vi "Psychro Solver.vi"(7 "Incomplete Air Flow State":T1={"Flow Rate [CFM]"=0.0, "Pressure [psia]"=14.696, "Dry Bulb Temp [DegF]"=-460.0, "Wet Bulb Temp [DegF]"=-460.0, "Relative Humidity [%]"=-460.0, "Humidity Ratio [lbmv/lbma]"=-460.0, "Grains [Gr/lbma]"=-460.0, "Specific Volume [ft^3/lbma]"=-460.0, "Enthalpy [BTU/lbm]"=-460.0, "Dew Point [DegF]"=-460.0}) -> (8 "Complete Air Flow State":T1={"Flow Rate [CFM]"=0.0, "Pressure [psia]"=0.0, "Dry Bulb Temp [DegF]"=-460.0, "Wet Bulb Temp [DegF]"=-460.0, "Relative Humidity [%]"=-460.0, "Humidity Ratio [lbmv/lbma]"=-460.0, "Grains [Gr/lbma]"=-460.0, "Specific Volume [ft^3/lbma]"=-460.0, "Enthalpy [BTU/lbm]"=-460.0, "Dew Point [DegF]"=-460.0})   [LabVIEW 2020]
uses:
  Utilities/Air Flow State.ctl
  Utilities/Air Constants.vi
panel:
  out "2nd Property":dbl
  out "1st Property":dbl
  out "2nd Known Index":u16(ring)=2 items=["DB", "WB", "RH", "HR", "Gr", "Vol", "h", "Dp"]
  out "array w/ 1st \nproperty set to -460":dbl[](array[numeric])=[-460.0, -460.0, -460.0, -460.0, -200.0, -460.0, -460.0, -460.0]
  out "array w/ subset deleted":dbl[](array[numeric])=[-460.0, -460.0, -460.0, -460.0, -200.0, -460.0, -460.0, -460.0]
  out "1st Known Index":u16(ring) items=["DB", "WB", "RH", "HR", "Gr", "Vol", "h", "Dp"]
  # "Data was generated using the the \nkW Psychrometric Functions Library for Excel:\n\nhttps://www.kw-engineering.com/psychrometrics/"
  # "As of 6/3/21 - Program is completed and checked with the following\nnotes:\n\n* CANNOT Perform Look-up if the two variables entered are:\n     DB & h\n     DB & v\n      h & v\n\n     This is because the excel function used to generate the tables MUST \n      have DB as one of the inputs, and the function cannot accept v or h as an input.\n\n*  Program does not behave well if input is WB & h. On psych chart, these two variables\n    appear to be independent (parallel lines)\n\n*Program does not behave well if input is HR/Gr & DP. On psych chart, these two variables\n     appear to be independent"
  # "These cases return NaN"
  # "TO DO: \n\nFigure out how to make program work for remaining scenarios\n\nDocument error range (a quick spot check never returned a value with more than 1% error. \nChecked for combinations compatible with the TRANE HDPsyChart App [must input DB]. Situations \nnot compatible with that App were checked by eye with the app's psych chart. P = 14.696 psia only\npressure checked so far.)"
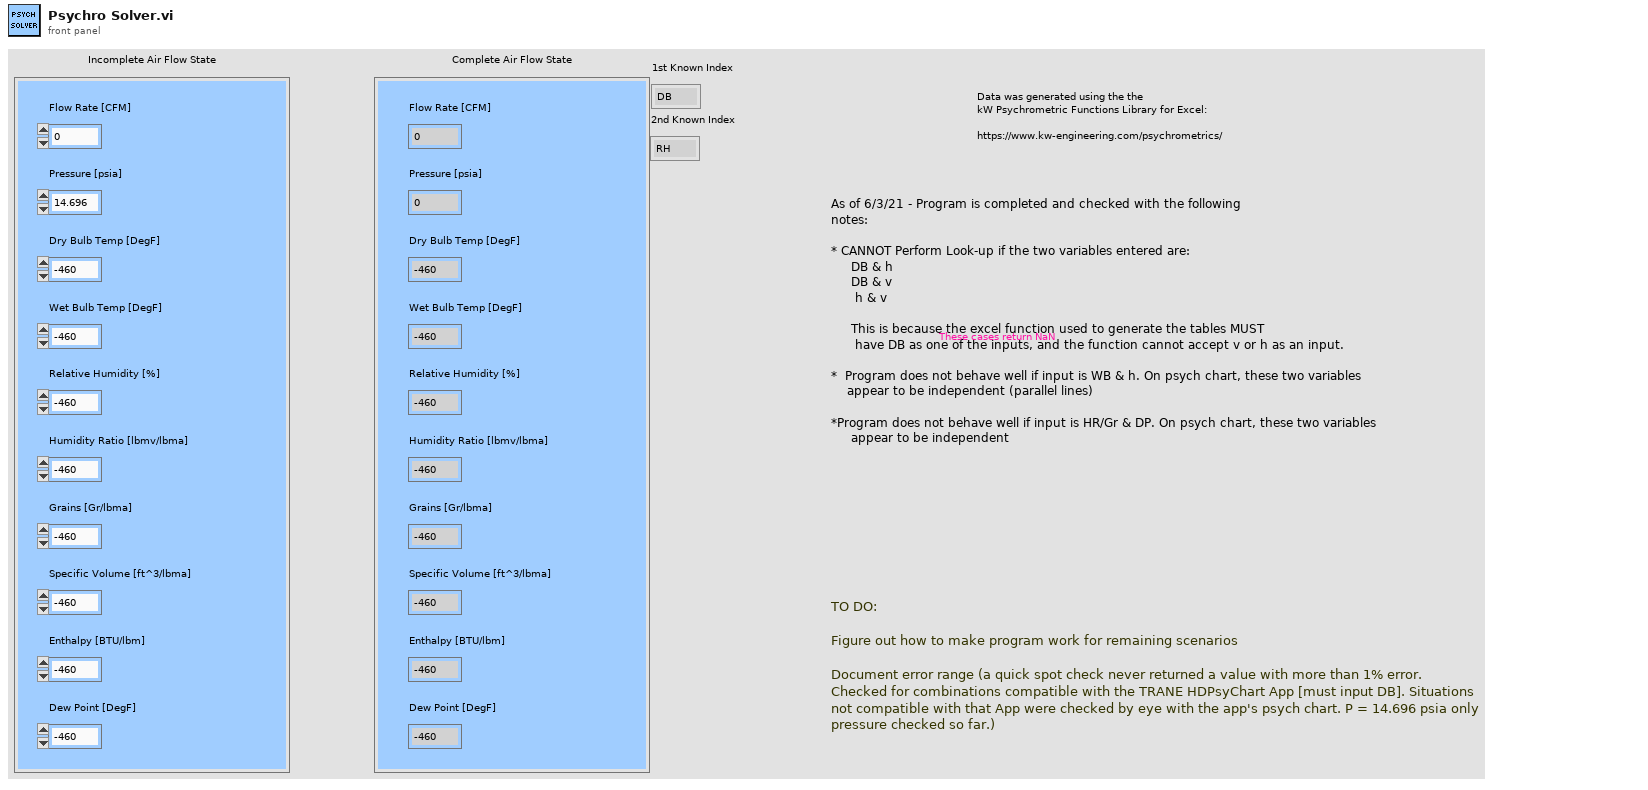
[diagram p1: front panel]
types:
  T1 = typedef "Air Flow State.ctl" = cluster{"Flow Rate [CFM]":dbl, "Pressure [psia]":dbl, "Dry Bulb Temp [DegF]":dbl, "Wet Bulb Temp [DegF]":dbl, "Relative Humidity [%]":dbl, "Humidity Ratio [lbmv/lbma]":dbl, "Grains [Gr/lbma]":dbl, "Specific Volume [ft^3/lbma]":dbl, "Enthalpy [BTU/lbm]":dbl, "Dew Point [DegF]":dbl}
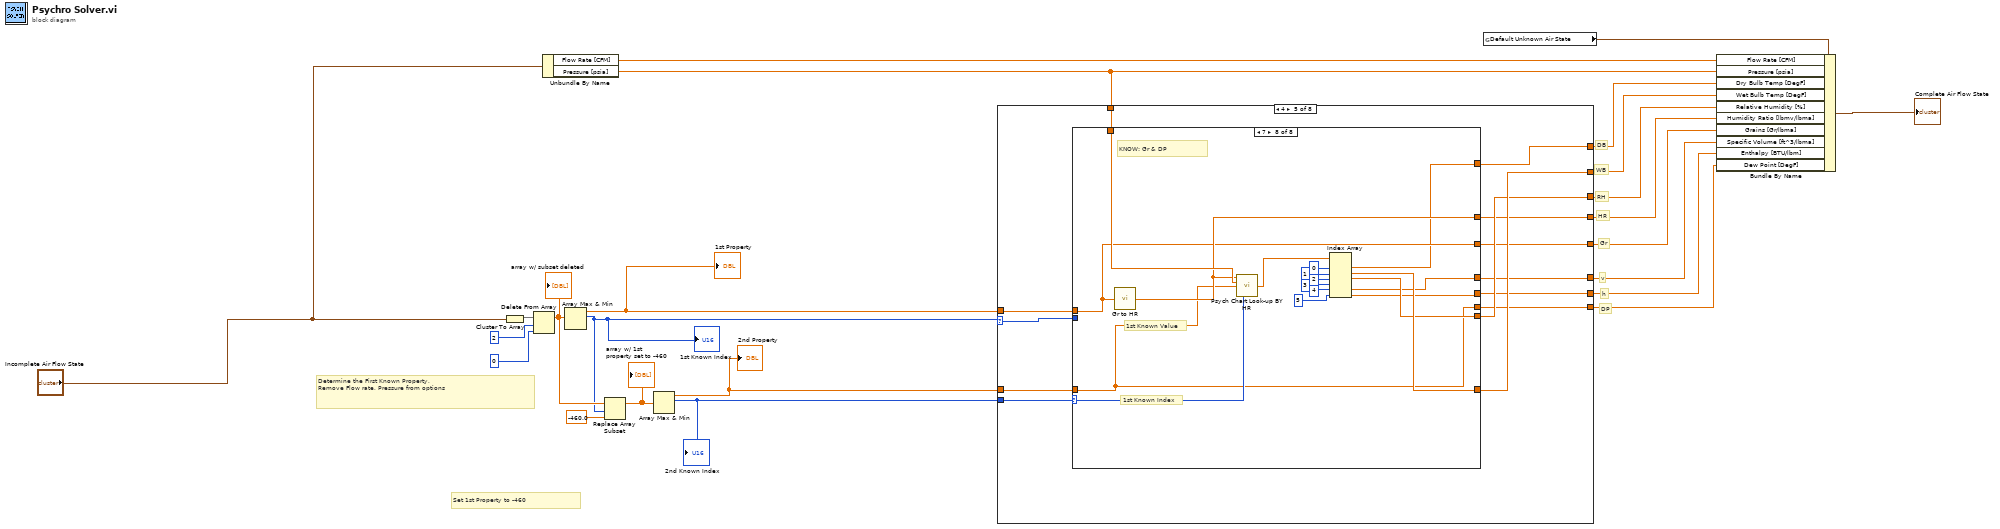
[diagram p0: block diagram]
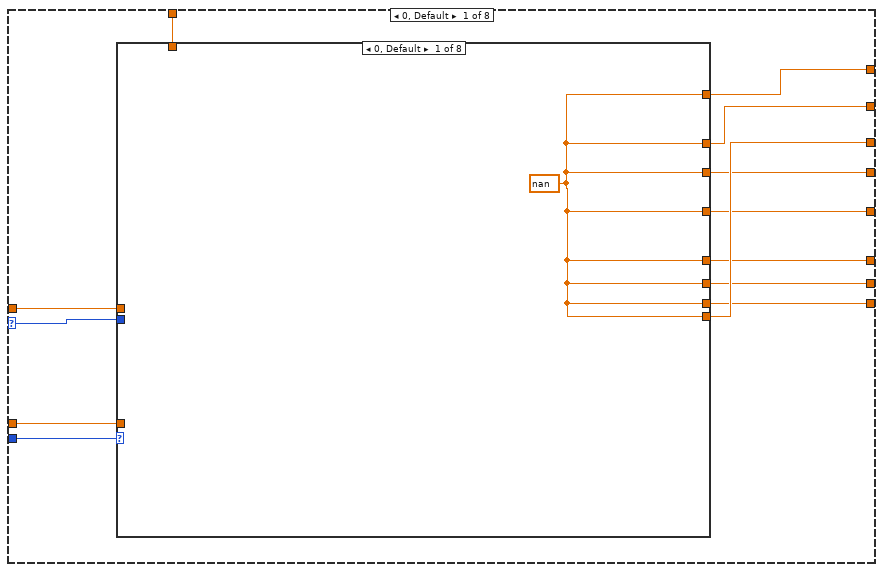
[diagram p2: hidden frame]
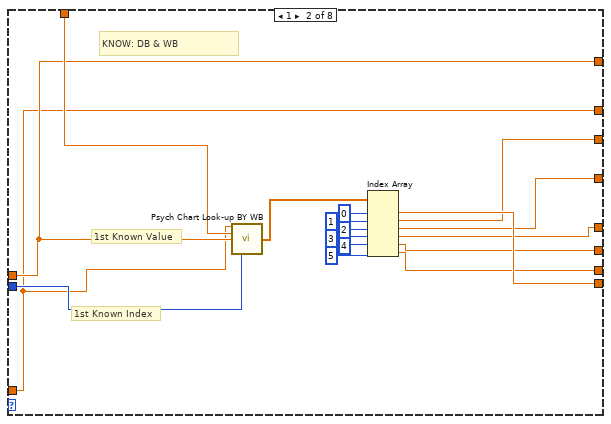
[diagram p3: hidden frame]
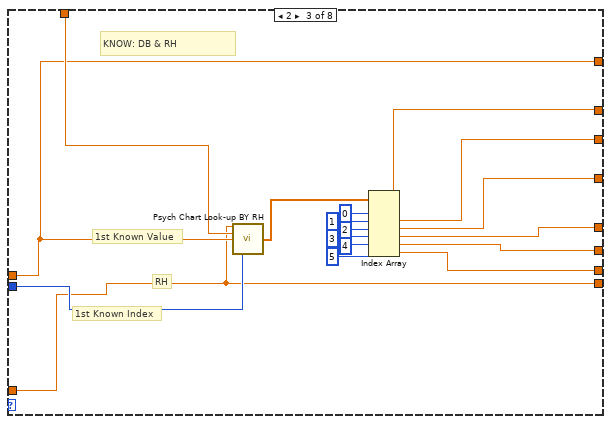
[diagram p4: hidden frame]
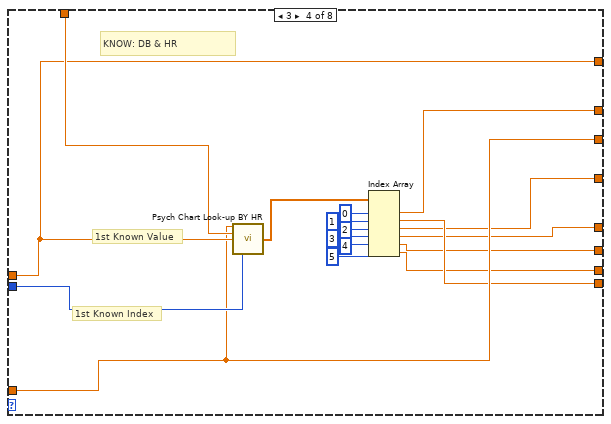
[diagram p5: hidden frame]
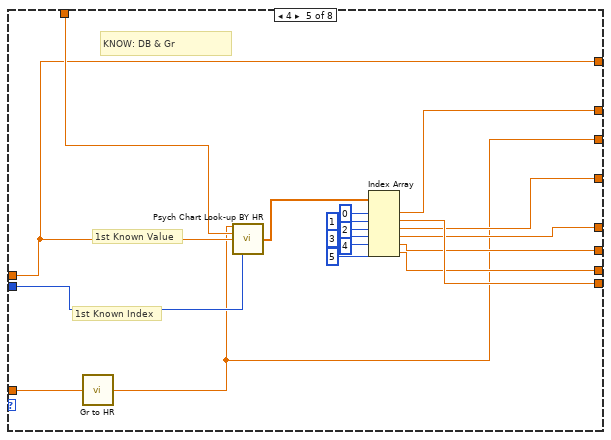
[diagram p6: hidden frame]
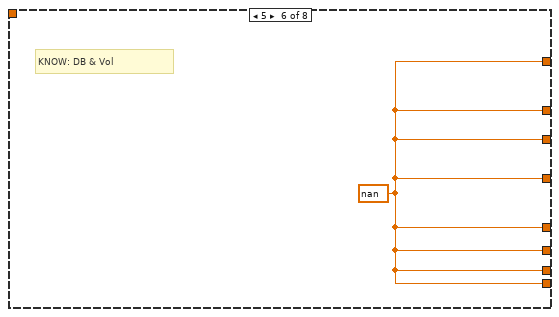
[diagram p7: hidden frame]
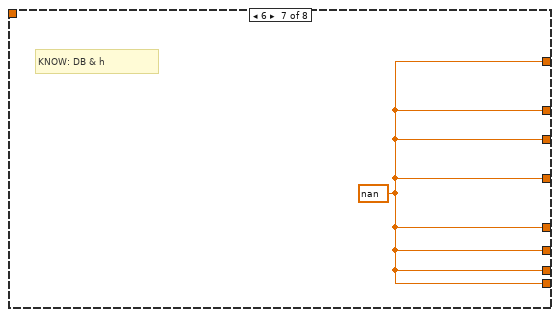
[diagram p8: hidden frame]
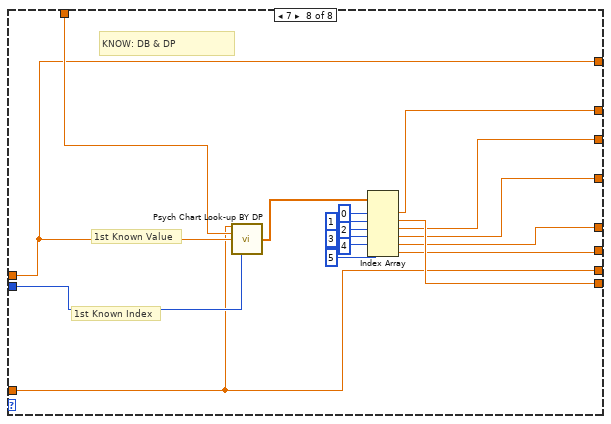
[diagram p9: hidden frame]
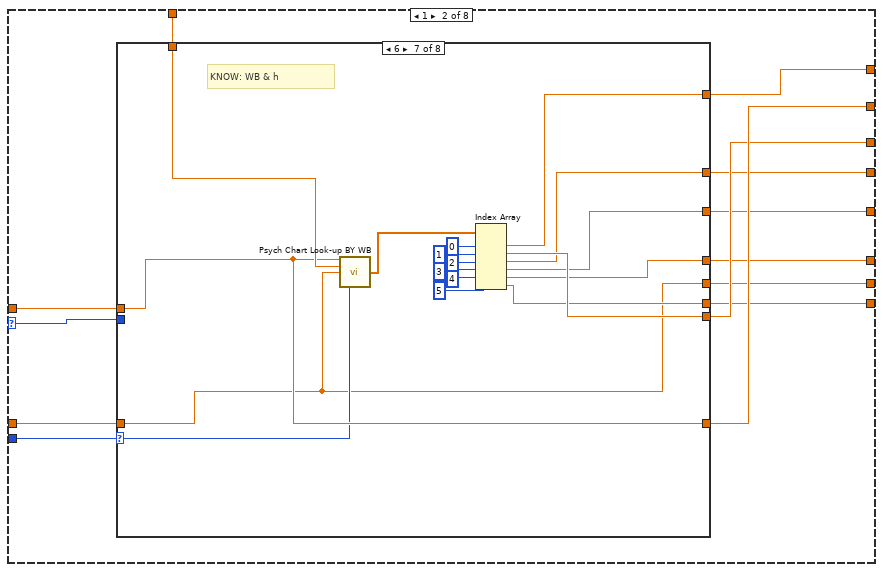
[diagram p10: hidden frame]
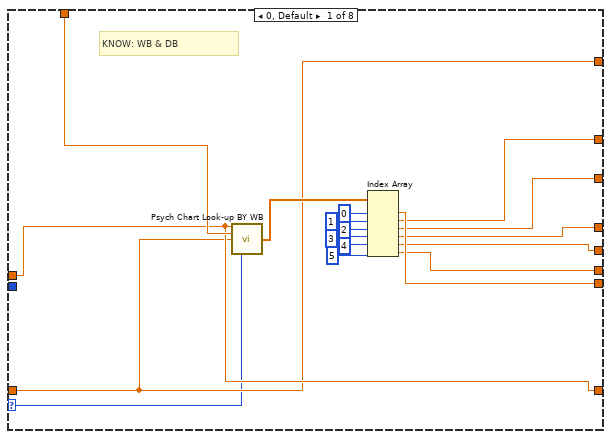
[diagram p11: hidden frame]
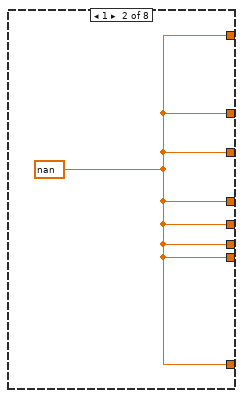
[diagram p12: hidden frame]
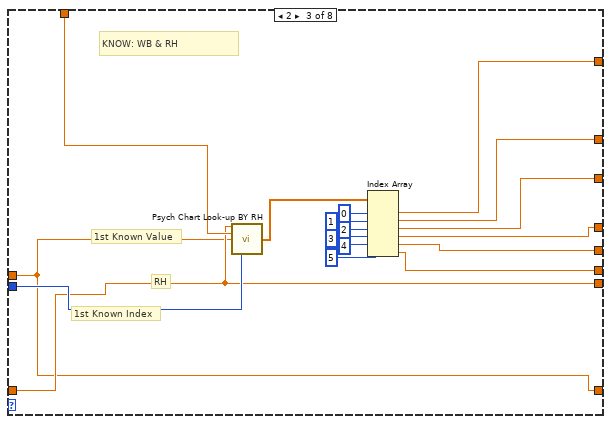
[diagram p13: hidden frame]
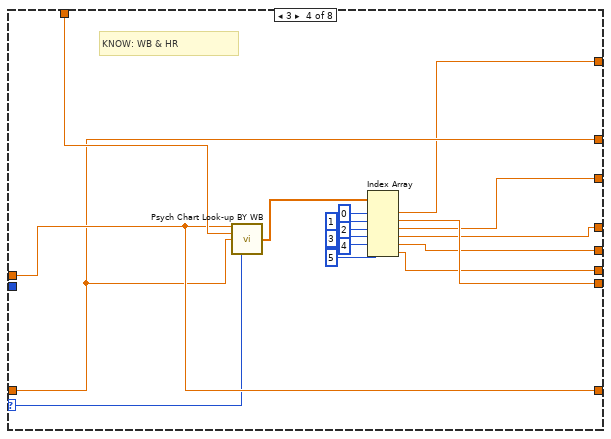
[diagram p14: hidden frame]
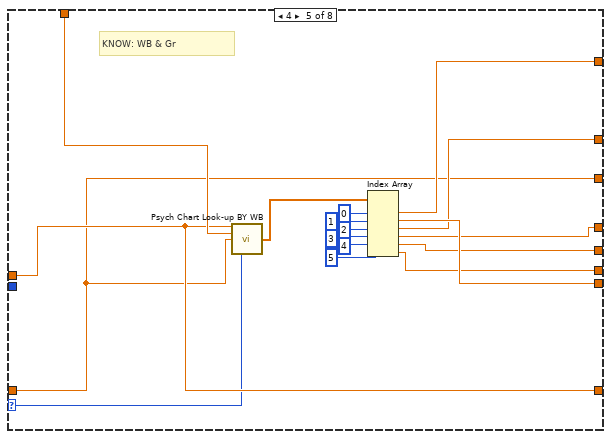
[diagram p15: hidden frame]
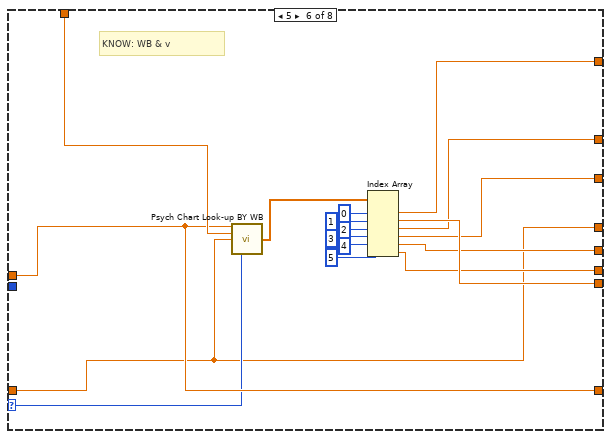
[diagram p16: hidden frame]
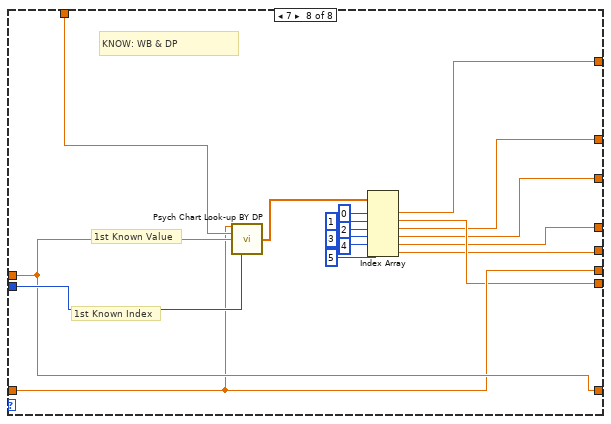
[diagram p17: hidden frame]
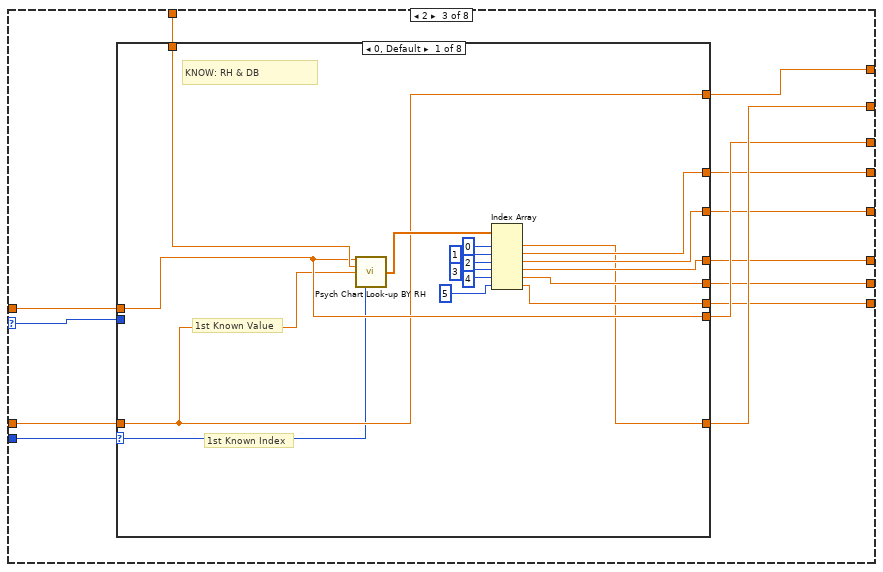
[diagram p18: hidden frame]
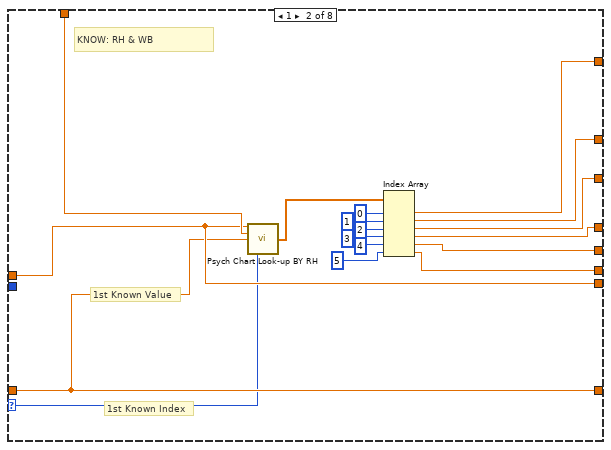
[diagram p19: hidden frame]
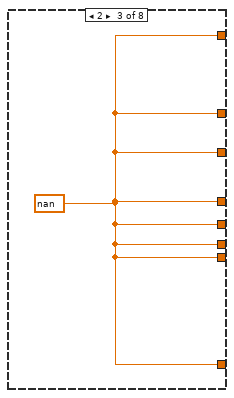
[diagram p20: hidden frame]
diagram:
  # "DP"
  # "h"
  # "v"
  # "Gr"
  # "HR"
  # "RH"
  # "WB"
  # "DB"
  # "Set 1st Property to -460"
  # "Determine the First Known Property, \nRemove Flow rate, Pressure from options"
  n1 = Cluster To Array(cluster="Incomplete Air Flow State") -> (array=w20:dbl[])
  n2 = Delete From Array(array=w20, length=2, index=0) -> (array with subset deleted=w17:dbl[])  [unwired: 1 out]
  "array w/ subset deleted" <- w17
  n3 = Unbundle By Name("Incomplete Air Flow State") -> ("Flow Rate [CFM]"=w10:dbl, "Pressure [psia]"=w9:dbl)
  n4 = Array Max & Min(array=w17) -> (max value=w12:dbl, max index (indices)=w14:i32)  [unwired: 2 out]
  "1st Known Index" <- w14
  "1st Property" <- w12
  n5 = Replace Array Subset(array=w17, new element=-460.0 ("new element/subarray"), index=w14) -> (w16:dbl[])
  "array w/ 1st \nproperty set to -460" <- w16
  n6 = Array Max & Min(array=w16) -> (max value=w11:dbl, max index (indices)=w13:i32)  [unwired: 2 out]
  "2nd Known Index" <- w13
  "2nd Property" <- w11
  n7 = case shown="4" w14 {
    selector: w14 -> [w36 w137 w270 w403 w520 w637 w738 w840]
    tunnel: w13 -> [w24 w138 w271 w404 w521 w638 w739 w828]
    tunnel: w12 -> [w35 w136 w269 w402 w519 w636 w737 w839]
    tunnel: w11 -> [w34 w135 w268 w401 w518 w635 w736 w838]
    tunnel: w9 -> [w33 w134 w267 w400 w517 w634 w735 w837]
    tunnel: [w32 w133 w266 w399 w516 w633 w734 w836] -> w8
    tunnel: [w31 w132 w265 w398 w515 w632 w733 w835] -> w7
    tunnel: [w30 w131 w264 w397 w514 w631 w732 w834] -> w6
    tunnel: [w29 w130 w263 w396 w513 w630 w731 w833] -> w5
    tunnel: [w28 w129 w262 w395 w512 w629 w730 w832] -> w4
    tunnel: [w27 w128 w261 w394 w511 w628 w729 w831] -> w3
    tunnel: [w26 w127 w260 w393 w510 w627 w728 w830] -> w2
    tunnel: [w25 w126 w259 w392 w509 w626 w727 w829] -> w1
    frame 0, Default {
      n8 = case shown="0, Default" w24 {
        tunnel: w36 -> [_ w53 w70 w87 w105 _ _ w124]
        tunnel: w35 -> [_ w52 w69 w86 w104 _ _ w123]
        tunnel: w34 -> [_ w45 w61 w77 w90 _ _ w109]
        tunnel: w33 -> [_ w54 w71 w88 w106 _ _ w125]
        tunnel: [w37 w52 w69 w86 w104 w107 w108 w123] -> w32
        tunnel: [w37 w45 w60 w78 w96 w107 w108 w115] -> w31
        tunnel: [w37 w44 w61 w76 w95 w107 w108 w114] -> w30
        tunnel: [w37 w43 w59 w77 w89 w107 w108 w113] -> w29
        tunnel: [w37 w42 w58 w75 w94 w107 w108 w112] -> w28
        tunnel: [w37 w41 w57 w74 w93 w107 w108 w111] -> w27
        tunnel: [w37 w40 w56 w73 w92 w107 w108 w110] -> w26
        tunnel: [w37 w38 w55 w72 w91 w107 w108 w109] -> w25
        frame 0, Default {
          w37 = nan
        }
        frame 1 {
          # "1st Known Index"
          # "1st Known Value"
          # "KNOW: DB & WB"
          n9 = call "Psych Chart Look-up BY WB.vi"("Wet Bulb Temp [DegF]"=w45, "Air Pressure [psia]"=w54, "1st known value"=w52, "1st Known Index"=w53) -> ("Output Array"=w46:dbl[])  [unwired: 11 in]
          n10 = Index Array(array=w46, index #1=0 ("index"), index #2=1 ("index"), index #3=2 ("index"), index #4=3 ("index"), index #5=4 ("index"), index #6=5 ("index")) -> (element #1=w44:dbl, element #2=w43:dbl, element #3=w42:dbl, element #4=w41:dbl, element #5=w40:dbl, element #6=w38:dbl)
        }
        frame 2 {
          # "RH"
          # "1st Known Index"
          # "1st Known Value"
          # "KNOW: DB & RH"
          n11 = call "Psych Chart Look-up BY RH.vi"("Relative Humidity [%]"=w61, "Air Pressure [psia]"=w71, "1st known value"=w69, "1st Known Index"=w70) -> ("Output Array"=w63:dbl[])  [unwired: 11 in]
          n12 = Index Array(array=w63, index #1=0 ("index"), index #2=1 ("index"), index #3=2 ("index"), index #4=3 ("index"), index #5=4 ("index"), index #6=5 ("index")) -> (element #1=w60:dbl, element #2=w59:dbl, element #3=w58:dbl, element #4=w57:dbl, element #5=w56:dbl, element #6=w55:dbl)
        }
        frame 3 {
          # "1st Known Index"
          # "1st Known Value"
          # "KNOW: DB & HR"
          n13 = call "Psych Chart Look-up BY HR.vi"("Humidity Ratio [-]"=w77, "Air Pressure [psia]"=w88, "1st known value"=w86, "1st Known Index"=w87) -> ("Output Array"=w80:dbl[])  [unwired: 11 in]
          n14 = Index Array(array=w80, index #1=0 ("index"), index #2=1 ("index"), index #3=2 ("index"), index #4=3 ("index"), index #5=4 ("index"), index #6=5 ("index")) -> (element #1=w78:dbl, element #2=w76:dbl, element #3=w75:dbl, element #4=w74:dbl, element #5=w73:dbl, element #6=w72:dbl)
        }
        frame 4 {
          # "1st Known Index"
          # "1st Known Value"
          # "KNOW: DB & Gr"
          n15 = call "Gr to HR.vi"("Grains [-]"=w90) -> ("Humidity Ratio [-]"=w89:dbl)
          n16 = call "Psych Chart Look-up BY HR.vi"("Humidity Ratio [-]"=w89, "Air Pressure [psia]"=w106, "1st known value"=w104, "1st Known Index"=w105) -> ("Output Array"=w98:dbl[])  [unwired: 11 in]
          n17 = Index Array(array=w98, index #1=0 ("index"), index #2=1 ("index"), index #3=2 ("index"), index #4=3 ("index"), index #5=4 ("index"), index #6=5 ("index")) -> (element #1=w96:dbl, element #2=w95:dbl, element #3=w94:dbl, element #4=w93:dbl, element #5=w92:dbl, element #6=w91:dbl)
        }
        frame 5 {
          w107 = nan
          # "KNOW: DB & Vol"
        }
        frame 6 {
          w108 = nan
          # "KNOW: DB & h"
        }
        frame 7 {
          # "1st Known Index"
          # "1st Known Value"
          # "KNOW: DB & DP"
          n18 = call "Psych Chart Look-up BY DP.vi"("Dew Point [DegF]"=w109, "Air Pressure [psia]"=w125, "1st known value"=w123, "1st Known Index"=w124) -> ("Output Array"=w117:dbl[])  [unwired: 11 in]
          n19 = Index Array(array=w117, index #1=0 ("index"), index #2=1 ("index"), index #3=2 ("index"), index #4=3 ("index"), index #5=4 ("index"), index #6=5 ("index")) -> (element #1=w115:dbl, element #2=w114:dbl, element #3=w113:dbl, element #4=w112:dbl, element #5=w111:dbl, element #6=w110:dbl)
        }
      }
    }
    frame 1 {
      n20 = case shown="6" w138 {
        selector: w138 -> [w146 _ _ w180 w198 w215 w232 _]
        tunnel: w137 -> [_ _ w172 _ _ _ _ w257]
        tunnel: w136 -> [w148 _ w164 w182 w199 w216 w233 w250]
        tunnel: w135 -> [w147 _ w165 w181 w191 w208 w225 w248]
        tunnel: w134 -> [w155 _ w173 w190 w207 w224 w241 w258]
        tunnel: [w147 w156 w162 w179 w197 w214 w231 w247] -> w133
        tunnel: [w148 w156 w164 w182 w199 w216 w233 w250] -> w132
        tunnel: [w145 w156 w165 w178 w196 w213 w230 w246] -> w131
        tunnel: [w144 w156 w161 w181 w192 w210 w228 w245] -> w130
        tunnel: [w143 w156 w160 w177 w191 w209 w227 w242] -> w129
        tunnel: [w142 w156 w159 w176 w195 w208 w226 w244] -> w128
        tunnel: [w141 w156 w158 w175 w194 w212 w225 w243] -> w127
        tunnel: [w139 w156 w157 w174 w193 w211 w229 w248] -> w126
        frame 0, Default {
          # "KNOW: WB & DB"
          n21 = call "Psych Chart Look-up BY WB.vi"("Wet Bulb Temp [DegF]"=w148, "Air Pressure [psia]"=w155, "1st known value"=w147, "1st Known Index"=w146) -> ("Output Array"=w149:dbl[])  [unwired: 11 in]
          n22 = Index Array(array=w149, index #1=0 ("index"), index #2=1 ("index"), index #3=2 ("index"), index #4=3 ("index"), index #5=4 ("index"), index #6=5 ("index")) -> (element #1=w145:dbl, element #2=w144:dbl, element #3=w143:dbl, element #4=w142:dbl, element #5=w141:dbl, element #6=w139:dbl)
        }
        frame 1 {
          w156 = nan
        }
        frame 2 {
          # "RH"
          # "1st Known Index"
          # "1st Known Value"
          # "KNOW: WB & RH"
          n23 = call "Psych Chart Look-up BY RH.vi"("Relative Humidity [%]"=w165, "Air Pressure [psia]"=w173, "1st known value"=w164, "1st Known Index"=w172) -> ("Output Array"=w166:dbl[])  [unwired: 11 in]
          n24 = Index Array(array=w166, index #1=0 ("index"), index #2=1 ("index"), index #3=2 ("index"), index #4=3 ("index"), index #5=4 ("index"), index #6=5 ("index")) -> (element #1=w162:dbl, element #2=w161:dbl, element #3=w160:dbl, element #4=w159:dbl, element #5=w158:dbl, element #6=w157:dbl)
        }
        frame 3 {
          # "KNOW: WB & HR"
          n25 = call "Psych Chart Look-up BY WB.vi"("Wet Bulb Temp [DegF]"=w182, "Air Pressure [psia]"=w190, "1st known value"=w181, "1st Known Index"=w180) -> ("Output Array"=w184:dbl[])  [unwired: 11 in]
          n26 = Index Array(array=w184, index #1=0 ("index"), index #2=1 ("index"), index #3=2 ("index"), index #4=3 ("index"), index #5=4 ("index"), index #6=5 ("index")) -> (element #1=w179:dbl, element #2=w178:dbl, element #3=w177:dbl, element #4=w176:dbl, element #5=w175:dbl, element #6=w174:dbl)
        }
        frame 4 {
          # "KNOW: WB & Gr"
          n27 = call "Psych Chart Look-up BY WB.vi"("Wet Bulb Temp [DegF]"=w199, "Air Pressure [psia]"=w207, "1st known value"=w191, "1st Known Index"=w198) -> ("Output Array"=w201:dbl[])  [unwired: 11 in]
          n28 = Index Array(array=w201, index #1=0 ("index"), index #2=1 ("index"), index #3=2 ("index"), index #4=3 ("index"), index #5=4 ("index"), index #6=5 ("index")) -> (element #1=w197:dbl, element #2=w196:dbl, element #3=w192:dbl, element #4=w195:dbl, element #5=w194:dbl, element #6=w193:dbl)
        }
        frame 5 {
          # "KNOW: WB & v"
          n29 = call "Psych Chart Look-up BY WB.vi"("Wet Bulb Temp [DegF]"=w216, "Air Pressure [psia]"=w224, "1st known value"=w208, "1st Known Index"=w215) -> ("Output Array"=w218:dbl[])  [unwired: 11 in]
          n30 = Index Array(array=w218, index #1=0 ("index"), index #2=1 ("index"), index #3=2 ("index"), index #4=3 ("index"), index #5=4 ("index"), index #6=5 ("index")) -> (element #1=w214:dbl, element #2=w213:dbl, element #3=w210:dbl, element #4=w209:dbl, element #5=w212:dbl, element #6=w211:dbl)
        }
        frame 6 {
          # "KNOW: WB & h"
          n31 = call "Psych Chart Look-up BY WB.vi"("Wet Bulb Temp [DegF]"=w233, "Air Pressure [psia]"=w241, "1st known value"=w225, "1st Known Index"=w232) -> ("Output Array"=w235:dbl[])  [unwired: 11 in]
          n32 = Index Array(array=w235, index #1=0 ("index"), index #2=1 ("index"), index #3=2 ("index"), index #4=3 ("index"), index #5=4 ("index"), index #6=5 ("index")) -> (element #1=w231:dbl, element #2=w230:dbl, element #3=w228:dbl, element #4=w227:dbl, element #5=w226:dbl, element #6=w229:dbl)
        }
        frame 7 {
          # "1st Known Index"
          # "1st Known Value"
          # "KNOW: WB & DP"
          n33 = call "Psych Chart Look-up BY DP.vi"("Dew Point [DegF]"=w248, "Air Pressure [psia]"=w258, "1st known value"=w250, "1st Known Index"=w257) -> ("Output Array"=w251:dbl[])  [unwired: 11 in]
          n34 = Index Array(array=w251, index #1=0 ("index"), index #2=1 ("index"), index #3=2 ("index"), index #4=3 ("index"), index #5=4 ("index"), index #6=5 ("index")) -> (element #1=w247:dbl, element #2=w246:dbl, element #3=w245:dbl, element #4=w242:dbl, element #5=w244:dbl, element #6=w243:dbl)
        }
      }
    }
    frame 2 {
      n35 = case shown="0, Default" w271 {
        selector: w271 -> [w272 w289 _ w307 w324 w341 w358 w375]
        tunnel: w270 -> [_ _ _ _ _ _ _ _]
        tunnel: w269 -> [w281 w298 _ w316 w333 w350 w367 w384]
        tunnel: w268 -> [w273 w296 _ w310 w326 w343 w360 w376]
        tunnel: w267 -> [w282 w299 _ w317 w334 w351 w368 w385]
        tunnel: [w273 w297 w306 w309 w328 w346 w364 w382] -> w266
        tunnel: [w274 w296 w306 w308 w327 w345 w363 w381] -> w265
        tunnel: [w281 w298 w306 w316 w333 w350 w367 w384] -> w264
        tunnel: [w280 w295 w306 w310 w325 w344 w362 w380] -> w263
        tunnel: [w279 w294 w306 w315 w326 w342 w361 w379] -> w262
        tunnel: [w278 w293 w306 w314 w332 w343 w359 w378] -> w261
        tunnel: [w277 w292 w306 w313 w331 w349 w360 w377] -> w260
        tunnel: [w275 w290 w306 w311 w329 w347 w365 w376] -> w259
        frame 0, Default {
          # "1st Known Index"
          # "1st Known Value"
          # "KNOW: RH & DB"
          n36 = call "Psych Chart Look-up BY RH.vi"("Relative Humidity [%]"=w281, "Air Pressure [psia]"=w282, "1st known value"=w273, "1st Known Index"=w272) -> ("Output Array"=w283:dbl[])  [unwired: 11 in]
          n37 = Index Array(array=w283, index #1=0 ("index"), index #2=1 ("index"), index #3=2 ("index"), index #4=3 ("index"), index #5=4 ("index"), index #6=5 ("index")) -> (element #1=w274:dbl, element #2=w280:dbl, element #3=w279:dbl, element #4=w278:dbl, element #5=w277:dbl, element #6=w275:dbl)
        }
        frame 1 {
          # "1st Known Index"
          # "1st Known Value"
          # "KNOW: RH & WB"
          n38 = call "Psych Chart Look-up BY RH.vi"("Relative Humidity [%]"=w298, "Air Pressure [psia]"=w299, "1st known value"=w296, "1st Known Index"=w289) -> ("Output Array"=w300:dbl[])  [unwired: 11 in]
          n39 = Index Array(array=w300, index #1=0 ("index"), index #2=1 ("index"), index #3=2 ("index"), index #4=3 ("index"), index #5=4 ("index"), index #6=5 ("index")) -> (element #1=w297:dbl, element #2=w295:dbl, element #3=w294:dbl, element #4=w293:dbl, element #5=w292:dbl, element #6=w290:dbl)
        }
        frame 2 {
          w306 = nan
        }
        frame 3 {
          # "1st Known Index"
          # "1st Known Value"
          # "KNOW: RH & HR"
          n40 = call "Psych Chart Look-up BY RH.vi"("Relative Humidity [%]"=w316, "Air Pressure [psia]"=w317, "1st known value"=w310, "1st Known Index"=w307) -> ("Output Array"=w318:dbl[])  [unwired: 11 in]
          n41 = Index Array(array=w318, index #1=0 ("index"), index #2=1 ("index"), index #3=2 ("index"), index #4=3 ("index"), index #5=4 ("index"), index #6=5 ("index")) -> (element #1=w309:dbl, element #2=w308:dbl, element #3=w315:dbl, element #4=w314:dbl, element #5=w313:dbl, element #6=w311:dbl)
        }
        frame 4 {
          # "1st Known Index"
          # "1st Known Value"
          # "KNOW: RH & Gr"
          n42 = call "Psych Chart Look-up BY RH.vi"("Relative Humidity [%]"=w333, "Air Pressure [psia]"=w334, "1st known value"=w326, "1st Known Index"=w324) -> ("Output Array"=w335:dbl[])  [unwired: 11 in]
          n43 = Index Array(array=w335, index #1=0 ("index"), index #2=1 ("index"), index #3=2 ("index"), index #4=3 ("index"), index #5=4 ("index"), index #6=5 ("index")) -> (element #1=w328:dbl, element #2=w327:dbl, element #3=w325:dbl, element #4=w332:dbl, element #5=w331:dbl, element #6=w329:dbl)
        }
        frame 5 {
          # "1st Known Index"
          # "1st Known Value"
          # "KNOW: RH & v"
          n44 = call "Psych Chart Look-up BY RH.vi"("Relative Humidity [%]"=w350, "Air Pressure [psia]"=w351, "1st known value"=w343, "1st Known Index"=w341) -> ("Output Array"=w352:dbl[])  [unwired: 11 in]
          n45 = Index Array(array=w352, index #1=0 ("index"), index #2=1 ("index"), index #3=2 ("index"), index #4=3 ("index"), index #5=4 ("index"), index #6=5 ("index")) -> (element #1=w346:dbl, element #2=w345:dbl, element #3=w344:dbl, element #4=w342:dbl, element #5=w349:dbl, element #6=w347:dbl)
        }
        frame 6 {
          # "1st Known Index"
          # "1st Known Value"
          # "KNOW: RH & h"
          n46 = call "Psych Chart Look-up BY RH.vi"("Relative Humidity [%]"=w367, "Air Pressure [psia]"=w368, "1st known value"=w360, "1st Known Index"=w358) -> ("Output Array"=w369:dbl[])  [unwired: 11 in]
          n47 = Index Array(array=w369, index #1=0 ("index"), index #2=1 ("index"), index #3=2 ("index"), index #4=3 ("index"), index #5=4 ("index"), index #6=5 ("index")) -> (element #1=w364:dbl, element #2=w363:dbl, element #3=w362:dbl, element #4=w361:dbl, element #5=w359:dbl, element #6=w365:dbl)
        }
        frame 7 {
          # "1st Known Index"
          # "1st Known Value"
          # "KNOW: RH & DP"
          n48 = call "Psych Chart Look-up BY RH.vi"("Relative Humidity [%]"=w384, "Air Pressure [psia]"=w385, "1st known value"=w376, "1st Known Index"=w375) -> ("Output Array"=w386:dbl[])  [unwired: 11 in]
          n49 = Index Array(array=w386, index #1=0 ("index"), index #2=1 ("index"), index #3=2 ("index"), index #4=3 ("index"), index #5=4 ("index"), index #6=5 ("index")) -> (element #1=w382:dbl, element #2=w381:dbl, element #3=w380:dbl, element #4=w379:dbl, element #5=w378:dbl, element #6=w377:dbl)
        }
      }
    }
    frame 3 {
      n50 = case shown="0, Default" w404 {
        selector: w404 -> [w405 w422 w439 _ _ w460 w477 w494]
        tunnel: w403 -> [_ _ _ _ _ _ _ _]
        tunnel: w402 -> [w407 w424 w441 _ _ w459 w476 w492]
        tunnel: w401 -> [w408 w430 w442 _ _ w462 w479 w495]
        tunnel: w400 -> [w415 w432 w449 _ _ w468 w485 w502]
        tunnel: [w408 w431 w448 w456 w457 w464 w482 w500] -> w399
        tunnel: [w409 w430 w442 w456 w457 w463 w481 w499] -> w398
        tunnel: [w406 w423 w440 w456 w457 w458 w475 w493] -> w397
        tunnel: [w407 w424 w441 w456 w457 w459 w476 w492] -> w396
        tunnel: [w414 w429 w447 w456 w457 w461 w480 w498] -> w395
        tunnel: [w413 w428 w446 w456 w457 w462 w478 w497] -> w394
        tunnel: [w412 w427 w445 w456 w457 w467 w479 w496] -> w393
        tunnel: [w410 w425 w443 w456 w457 w465 w483 w495] -> w392
        frame 0, Default {
          # "1st Known Index"
          # "1st Known Value"
          # "KNOW: HR & DB"
          n51 = call "Psych Chart Look-up BY HR.vi"("Humidity Ratio [-]"=w407, "Air Pressure [psia]"=w415, "1st known value"=w408, "1st Known Index"=w405) -> ("Output Array"=w416:dbl[])  [unwired: 11 in]
          n52 = Index Array(array=w416, index #1=0 ("index"), index #2=1 ("index"), index #3=2 ("index"), index #4=3 ("index"), index #5=4 ("index"), index #6=5 ("index")) -> (element #1=w409:dbl, element #2=w406:dbl, element #3=w414:dbl, element #4=w413:dbl, element #5=w412:dbl, element #6=w410:dbl)
        }
        frame 1 {
          # "1st Known Index"
          # "1st Known Value"
          # "KNOW: HR & WB"
          n53 = call "Psych Chart Look-up BY HR.vi"("Humidity Ratio [-]"=w424, "Air Pressure [psia]"=w432, "1st known value"=w430, "1st Known Index"=w422) -> ("Output Array"=w433:dbl[])  [unwired: 11 in]
          n54 = Index Array(array=w433, index #1=0 ("index"), index #2=1 ("index"), index #3=2 ("index"), index #4=3 ("index"), index #5=4 ("index"), index #6=5 ("index")) -> (element #1=w431:dbl, element #2=w423:dbl, element #3=w429:dbl, element #4=w428:dbl, element #5=w427:dbl, element #6=w425:dbl)
        }
        frame 2 {
          # "1st Known Index"
          # "1st Known Value"
          # "KNOW: HR & RH"
          n55 = call "Psych Chart Look-up BY RH.vi"("Relative Humidity [%]"=w442, "Air Pressure [psia]"=w449, "1st known value"=w441, "1st Known Index"=w439) -> ("Output Array"=w450:dbl[])  [unwired: 11 in]
          n56 = Index Array(array=w450, index #1=0 ("index"), index #2=1 ("index"), index #3=2 ("index"), index #4=3 ("index"), index #5=4 ("index"), index #6=5 ("index")) -> (element #1=w448:dbl, element #2=w440:dbl, element #3=w447:dbl, element #4=w446:dbl, element #5=w445:dbl, element #6=w443:dbl)
        }
        frame 3 {
          w456 = nan
        }
        frame 4 {
          w457 = nan
          # "GRAINS AND HR ARE NOT INDEPENDENT\nSTATE VARIABLES"
        }
        frame 5 {
          # "1st Known Index"
          # "1st Known Value"
          # "KNOW: HR & v"
          n57 = call "Psych Chart Look-up BY HR.vi"("Humidity Ratio [-]"=w459, "Air Pressure [psia]"=w468, "1st known value"=w462, "1st Known Index"=w460) -> ("Output Array"=w469:dbl[])  [unwired: 11 in]
          n58 = Index Array(array=w469, index #1=0 ("index"), index #2=1 ("index"), index #3=2 ("index"), index #4=3 ("index"), index #5=4 ("index"), index #6=5 ("index")) -> (element #1=w464:dbl, element #2=w463:dbl, element #3=w458:dbl, element #4=w461:dbl, element #5=w467:dbl, element #6=w465:dbl)
        }
        frame 6 {
          # "1st Known Index"
          # "1st Known Value"
          # "KNOW: HR & h"
          n59 = call "Psych Chart Look-up BY HR.vi"("Humidity Ratio [-]"=w476, "Air Pressure [psia]"=w485, "1st known value"=w479, "1st Known Index"=w477) -> ("Output Array"=w486:dbl[])  [unwired: 11 in]
          n60 = Index Array(array=w486, index #1=0 ("index"), index #2=1 ("index"), index #3=2 ("index"), index #4=3 ("index"), index #5=4 ("index"), index #6=5 ("index")) -> (element #1=w482:dbl, element #2=w481:dbl, element #3=w475:dbl, element #4=w480:dbl, element #5=w478:dbl, element #6=w483:dbl)
        }
        frame 7 {
          # "1st Known Index"
          # "1st Known Value"
          # "KNOW: HR & DP"
          n61 = call "Psych Chart Look-up BY HR.vi"("Humidity Ratio [-]"=w492, "Air Pressure [psia]"=w502, "1st known value"=w495, "1st Known Index"=w494) -> ("Output Array"=w503:dbl[])  [unwired: 11 in]
          n62 = Index Array(array=w503, index #1=0 ("index"), index #2=1 ("index"), index #3=2 ("index"), index #4=3 ("index"), index #5=4 ("index"), index #6=5 ("index")) -> (element #1=w500:dbl, element #2=w499:dbl, element #3=w493:dbl, element #4=w498:dbl, element #5=w497:dbl, element #6=w496:dbl)
        }
      }
    }
    frame 4 {
      n63 = case shown="7" w521 {
        selector: w521 -> [w524 w543 _ _ _ w580 w597 w615]
        tunnel: w520 -> [_ _ w559 _ _ _ _ _]
        tunnel: w519 -> [w525 w544 w560 _ _ w581 w598 w616]
        tunnel: w518 -> [w528 w540 w558 _ _ w577 w592 w610]
        tunnel: w517 -> [w532 w549 w566 _ _ w585 w602 w619]
        tunnel: [w528 w539 w561 w573 w574 w578 w596 w614] -> w516
        tunnel: [w529 w540 w557 w573 w574 w576 w595 w613] -> w515
        tunnel: [w527 w546 w558 w573 w574 w575 w594 w612] -> w514
        tunnel: [w526 w545 w556 w573 w574 w582 w599 w617] -> w513
        tunnel: [w525 w544 w560 w573 w574 w581 w598 w616] -> w512
        tunnel: [w523 w542 w563 w573 w574 w577 w593 w611] -> w511
        tunnel: [w522 w541 w562 w573 w574 w579 w592 w609] -> w510
        tunnel: [w530 w547 w564 w573 w574 w583 w600 w610] -> w509
        frame 0, Default {
          # "1st Known Index"
          # "1st Known Value"
          # "KNOW: Gr & DB"
          n64 = call "Gr to HR.vi"("Grains [-]"=w525) -> ("Humidity Ratio [-]"=w526:dbl)
          n65 = call "Psych Chart Look-up BY HR.vi"("Humidity Ratio [-]"=w526, "Air Pressure [psia]"=w532, "1st known value"=w528, "1st Known Index"=w524) -> ("Output Array"=w533:dbl[])  [unwired: 11 in]
          n66 = Index Array(array=w533, index #1=0 ("index"), index #2=1 ("index"), index #3=2 ("index"), index #4=3 ("index"), index #5=4 ("index"), index #6=5 ("index")) -> (element #1=w529:dbl, element #2=w527:dbl, element #4=w523:dbl, element #5=w522:dbl, element #6=w530:dbl)  [unwired: 1 out]
        }
        frame 1 {
          # "1st Known Index"
          # "1st Known Value"
          # "KNOW: Gr & WB"
          n67 = call "Gr to HR.vi"("Grains [-]"=w544) -> ("Humidity Ratio [-]"=w545:dbl)
          n68 = call "Psych Chart Look-up BY HR.vi"("Humidity Ratio [-]"=w545, "Air Pressure [psia]"=w549, "1st known value"=w540, "1st Known Index"=w543) -> ("Output Array"=w550:dbl[])  [unwired: 11 in]
          n69 = Index Array(array=w550, index #1=0 ("index"), index #2=1 ("index"), index #3=2 ("index"), index #4=3 ("index"), index #5=4 ("index"), index #6=5 ("index")) -> (element #1=w539:dbl, element #2=w546:dbl, element #4=w542:dbl, element #5=w541:dbl, element #6=w547:dbl)  [unwired: 1 out]
        }
        frame 2 {
          # "1st Known Index"
          # "1st Known Value"
          # "KNOW: Gr & RH"
          n70 = call "Psych Chart Look-up BY RH.vi"("Relative Humidity [%]"=w558, "Air Pressure [psia]"=w566, "1st known value"=w560, "1st Known Index"=w559) -> ("Output Array"=w567:dbl[])  [unwired: 11 in]
          n71 = Index Array(array=w567, index #1=0 ("index"), index #2=1 ("index"), index #3=2 ("index"), index #4=3 ("index"), index #5=4 ("index"), index #6=5 ("index")) -> (element #1=w561:dbl, element #2=w557:dbl, element #3=w556:dbl, element #4=w563:dbl, element #5=w562:dbl, element #6=w564:dbl)
        }
        frame 3 {
          w573 = nan
          # "GRAINS AND HR ARE NOT INDEPENDENT\nSTATE VARIABLES"
        }
        frame 4 {
          w574 = nan
        }
        frame 5 {
          # "1st Known Index"
          # "1st Known Value"
          # "KNOW: Gr & v"
          n72 = call "Gr to HR.vi"("Grains [-]"=w581) -> ("Humidity Ratio [-]"=w582:dbl)
          n73 = call "Psych Chart Look-up BY HR.vi"("Humidity Ratio [-]"=w582, "Air Pressure [psia]"=w585, "1st known value"=w577, "1st Known Index"=w580) -> ("Output Array"=w586:dbl[])  [unwired: 11 in]
          n74 = Index Array(array=w586, index #1=0 ("index"), index #2=1 ("index"), index #3=2 ("index"), index #4=3 ("index"), index #5=4 ("index"), index #6=5 ("index")) -> (element #1=w578:dbl, element #2=w576:dbl, element #3=w575:dbl, element #5=w579:dbl, element #6=w583:dbl)  [unwired: 1 out]
        }
        frame 6 {
          # "1st Known Index"
          # "1st Known Value"
          # "KNOW: Gr & h"
          n75 = call "Gr to HR.vi"("Grains [-]"=w598) -> ("Humidity Ratio [-]"=w599:dbl)
          n76 = call "Psych Chart Look-up BY HR.vi"("Humidity Ratio [-]"=w599, "Air Pressure [psia]"=w602, "1st known value"=w592, "1st Known Index"=w597) -> ("Output Array"=w603:dbl[])  [unwired: 11 in]
          n77 = Index Array(array=w603, index #1=0 ("index"), index #2=1 ("index"), index #3=2 ("index"), index #4=3 ("index"), index #5=4 ("index"), index #6=5 ("index")) -> (element #1=w596:dbl, element #2=w595:dbl, element #3=w594:dbl, element #5=w593:dbl, element #6=w600:dbl)  [unwired: 1 out]
        }
        frame 7 {
          # "1st Known Index"
          # "1st Known Value"
          # "KNOW: Gr & DP"
          n78 = call "Gr to HR.vi"("Grains [-]"=w616) -> ("Humidity Ratio [-]"=w617:dbl)
          n79 = call "Psych Chart Look-up BY HR.vi"("Humidity Ratio [-]"=w617, "Air Pressure [psia]"=w619, "1st known value"=w610, "1st Known Index"=w615) -> ("Output Array"=w620:dbl[])  [unwired: 11 in]
          n80 = Index Array(array=w620, index #1=0 ("index"), index #2=1 ("index"), index #3=2 ("index"), index #4=3 ("index"), index #5=4 ("index"), index #6=5 ("index")) -> (element #1=w614:dbl, element #2=w613:dbl, element #3=w612:dbl, element #5=w611:dbl, element #6=w609:dbl)  [unwired: 1 out]
        }
      }
    }
    frame 5 {
      n81 = case shown="0, Default" w638 {
        tunnel: w637 -> [_ w644 w662 w679 w696 _ _ w713]
        tunnel: w636 -> [_ w640 w659 w677 w693 _ _ w710]
        tunnel: w635 -> [_ w643 w657 w675 w691 _ _ w714]
        tunnel: w634 -> [_ w650 w667 w684 w701 _ _ w720]
        tunnel: [w639 w645 w663 w680 w697 w708 w709 w718] -> w633
        tunnel: [w639 w643 w658 w676 w695 w708 w709 w717] -> w632
        tunnel: [w639 w647 w657 w674 w694 w708 w709 w716] -> w631
        tunnel: [w639 w642 w661 w675 w692 w708 w709 w712] -> w630
        tunnel: [w639 w641 w660 w678 w691 w708 w709 w711] -> w629
        tunnel: [w639 w640 w659 w677 w693 w708 w709 w710] -> w628
        tunnel: [w639 w646 w664 w681 w698 w708 w709 w715] -> w627
        tunnel: [w639 w648 w665 w682 w699 w708 w709 w714] -> w626
        frame 0, Default {
          w639 = nan
          # "No Independent table for v"
        }
        frame 1 {
          # "1st Known Index"
          # "1st Known Value"
          # "KNOW: v & WB"
          n82 = call "Psych Chart Look-up BY WB.vi"("Wet Bulb Temp [DegF]"=w643, "Air Pressure [psia]"=w650, "1st known value"=w640, "1st Known Index"=w644) -> ("Output Array"=w651:dbl[])  [unwired: 11 in]
          n83 = Index Array(array=w651, index #1=0 ("index"), index #2=1 ("index"), index #3=2 ("index"), index #4=3 ("index"), index #5=4 ("index"), index #6=5 ("index")) -> (element #1=w645:dbl, element #2=w647:dbl, element #3=w642:dbl, element #4=w641:dbl, element #5=w646:dbl, element #6=w648:dbl)
        }
        frame 2 {
          # "1st Known Index"
          # "1st Known Value"
          # "KNOW: v & RH"
          n84 = call "Psych Chart Look-up BY RH.vi"("Relative Humidity [%]"=w657, "Air Pressure [psia]"=w667, "1st known value"=w659, "1st Known Index"=w662) -> ("Output Array"=w668:dbl[])  [unwired: 11 in]
          n85 = Index Array(array=w668, index #1=0 ("index"), index #2=1 ("index"), index #3=2 ("index"), index #4=3 ("index"), index #5=4 ("index"), index #6=5 ("index")) -> (element #1=w663:dbl, element #2=w658:dbl, element #3=w661:dbl, element #4=w660:dbl, element #5=w664:dbl, element #6=w665:dbl)
        }
        frame 3 {
          # "1st Known Index"
          # "1st Known Value"
          # "KNOW: v & HR"
          n86 = call "Psych Chart Look-up BY HR.vi"("Humidity Ratio [-]"=w675, "Air Pressure [psia]"=w684, "1st known value"=w677, "1st Known Index"=w679) -> ("Output Array"=w685:dbl[])  [unwired: 11 in]
          n87 = Index Array(array=w685, index #1=0 ("index"), index #2=1 ("index"), index #3=2 ("index"), index #4=3 ("index"), index #5=4 ("index"), index #6=5 ("index")) -> (element #1=w680:dbl, element #2=w676:dbl, element #3=w674:dbl, element #4=w678:dbl, element #5=w681:dbl, element #6=w682:dbl)
        }
        frame 4 {
          # "1st Known Index"
          # "1st Known Value"
          # "KNOW: v & Gr"
          n88 = call "Gr to HR.vi"("Grains [-]"=w691) -> ("Humidity Ratio [-]"=w692:dbl)
          n89 = call "Psych Chart Look-up BY HR.vi"("Humidity Ratio [-]"=w692, "Air Pressure [psia]"=w701, "1st known value"=w693, "1st Known Index"=w696) -> ("Output Array"=w702:dbl[])  [unwired: 11 in]
          n90 = Index Array(array=w702, index #1=0 ("index"), index #2=1 ("index"), index #3=2 ("index"), index #4=3 ("index"), index #5=4 ("index"), index #6=5 ("index")) -> (element #1=w697:dbl, element #2=w695:dbl, element #3=w694:dbl, element #5=w698:dbl, element #6=w699:dbl)  [unwired: 1 out]
        }
        frame 5 {
          w708 = nan
        }
        frame 6 {
          w709 = nan
          # "6/3/21: Do not have a dataset\norganized by volume or enthalpy\n(did not exist in source function)"
        }
        frame 7 {
          # "1st Known Index"
          # "1st Known Value"
          # "KNOW: v & DP"
          n91 = call "Psych Chart Look-up BY DP.vi"("Dew Point [DegF]"=w714, "Air Pressure [psia]"=w720, "1st known value"=w710, "1st Known Index"=w713) -> ("Output Array"=w721:dbl[])  [unwired: 11 in]
          n92 = Index Array(array=w721, index #1=0 ("index"), index #2=1 ("index"), index #3=2 ("index"), index #4=3 ("index"), index #5=4 ("index"), index #6=5 ("index")) -> (element #1=w718:dbl, element #2=w717:dbl, element #3=w716:dbl, element #4=w712:dbl, element #5=w711:dbl, element #6=w715:dbl)
        }
      }
    }
    frame 6 {
      n93 = case shown="0, Default" w739 {
        tunnel: w738 -> [_ w746 w764 w781 w798 _ _ w815]
        tunnel: w737 -> [_ w742 w761 w779 w793 _ _ w812]
        tunnel: w736 -> [_ w745 w758 w775 w794 _ _ w816]
        tunnel: w735 -> [_ w751 w768 w785 w802 _ _ w821]
        tunnel: [w740 w747 w765 w782 w799 w809 w810 w819] -> w734
        tunnel: [w740 w745 w759 w777 w797 w809 w810 w818] -> w733
        tunnel: [w740 w748 w758 w776 w796 w809 w810 w817] -> w732
        tunnel: [w740 w744 w763 w775 w795 w809 w810 w814] -> w731
        tunnel: [w740 w743 w762 w780 w794 w809 w810 w813] -> w730
        tunnel: [w740 w741 w760 w778 w792 w809 w810 w811] -> w729
        tunnel: [w740 w742 w761 w779 w793 w809 w810 w812] -> w728
        tunnel: [w740 w749 w766 w783 w800 w809 w810 w816] -> w727
        frame 0, Default {
          w740 = nan
          # "No Independent table for h"
        }
        frame 1 {
          # "1st Known Index"
          # "1st Known Value"
          # "KNOW: h & WB"
          n94 = call "Psych Chart Look-up BY WB.vi"("Wet Bulb Temp [DegF]"=w745, "Air Pressure [psia]"=w751, "1st known value"=w742, "1st Known Index"=w746) -> ("Output Array"=w752:dbl[])  [unwired: 11 in]
          n95 = Index Array(array=w752, index #1=0 ("index"), index #2=1 ("index"), index #3=2 ("index"), index #4=3 ("index"), index #5=4 ("index"), index #6=5 ("index")) -> (element #1=w747:dbl, element #2=w748:dbl, element #3=w744:dbl, element #4=w743:dbl, element #5=w741:dbl, element #6=w749:dbl)
        }
        frame 2 {
          # "1st Known Index"
          # "1st Known Value"
          # "KNOW: h & RH"
          n96 = call "Psych Chart Look-up BY RH.vi"("Relative Humidity [%]"=w758, "Air Pressure [psia]"=w768, "1st known value"=w761, "1st Known Index"=w764) -> ("Output Array"=w769:dbl[])  [unwired: 11 in]
          n97 = Index Array(array=w769, index #1=0 ("index"), index #2=1 ("index"), index #3=2 ("index"), index #4=3 ("index"), index #5=4 ("index"), index #6=5 ("index")) -> (element #1=w765:dbl, element #2=w759:dbl, element #3=w763:dbl, element #4=w762:dbl, element #5=w760:dbl, element #6=w766:dbl)
        }
        frame 3 {
          # "1st Known Index"
          # "1st Known Value"
          # "KNOW: h & HR"
          n98 = call "Psych Chart Look-up BY HR.vi"("Humidity Ratio [-]"=w775, "Air Pressure [psia]"=w785, "1st known value"=w779, "1st Known Index"=w781) -> ("Output Array"=w786:dbl[])  [unwired: 11 in]
          n99 = Index Array(array=w786, index #1=0 ("index"), index #2=1 ("index"), index #3=2 ("index"), index #4=3 ("index"), index #5=4 ("index"), index #6=5 ("index")) -> (element #1=w782:dbl, element #2=w777:dbl, element #3=w776:dbl, element #4=w780:dbl, element #5=w778:dbl, element #6=w783:dbl)
        }
        frame 4 {
          # "1st Known Index"
          # "1st Known Value"
          # "KNOW: h & Gr"
          n100 = call "Gr to HR.vi"("Grains [-]"=w794) -> ("Humidity Ratio [-]"=w795:dbl)
          n101 = call "Psych Chart Look-up BY HR.vi"("Humidity Ratio [-]"=w795, "Air Pressure [psia]"=w802, "1st known value"=w793, "1st Known Index"=w798) -> ("Output Array"=w803:dbl[])  [unwired: 11 in]
          n102 = Index Array(array=w803, index #1=0 ("index"), index #2=1 ("index"), index #3=2 ("index"), index #4=3 ("index"), index #5=4 ("index"), index #6=5 ("index")) -> (element #1=w799:dbl, element #2=w797:dbl, element #3=w796:dbl, element #5=w792:dbl, element #6=w800:dbl)  [unwired: 1 out]
        }
        frame 5 {
          w809 = nan
          # "6/3/21: Do not have a dataset\norganized by volume or enthalpy\n(did not exist in source function)"
        }
        frame 6 {
          w810 = nan
          # "DNE"
        }
        frame 7 {
          # "1st Known Index"
          # "1st Known Value"
          # "KNOW: h & DP"
          n103 = call "Psych Chart Look-up BY DP.vi"("Dew Point [DegF]"=w816, "Air Pressure [psia]"=w821, "1st known value"=w812, "1st Known Index"=w815) -> ("Output Array"=w822:dbl[])  [unwired: 11 in]
          n104 = Index Array(array=w822, index #1=0 ("index"), index #2=1 ("index"), index #3=2 ("index"), index #4=3 ("index"), index #5=4 ("index"), index #6=5 ("index")) -> (element #1=w819:dbl, element #2=w818:dbl, element #3=w817:dbl, element #4=w814:dbl, element #5=w813:dbl, element #6=w811:dbl)
        }
      }
    }
    frame 7 {
      n105 = case shown="0, Default" w828 {
        selector: w828 -> [w843 w861 w879 w897 w915 w933 w951 _]
        tunnel: w840 -> [_ _ _ _ _ _ _ _]
        tunnel: w839 -> [w841 w860 w878 w896 w914 w932 w950 _]
        tunnel: w838 -> [w842 w859 w875 w893 w910 w927 w943 _]
        tunnel: w837 -> [w857 w874 w891 w908 w925 w942 w959 _]
        tunnel: [w842 w858 w877 w895 w913 w931 w949 w960] -> w836
        tunnel: [w849 w859 w876 w894 w912 w930 w948 w960] -> w835
        tunnel: [w848 w866 w875 w892 w911 w929 w947 w960] -> w834
        tunnel: [w847 w865 w883 w893 w909 w928 w946 w960] -> w833
        tunnel: [w846 w864 w882 w900 w910 w926 w945 w960] -> w832
        tunnel: [w845 w863 w881 w899 w917 w927 w944 w960] -> w831
        tunnel: [w844 w862 w880 w898 w916 w934 w943 w960] -> w830
        tunnel: [w841 w860 w878 w896 w914 w932 w950 w960] -> w829
        frame 0, Default {
          # "1st Known Index"
          # "1st Known Value"
          # "KNOW: DP & DB"
          n106 = call "Psych Chart Look-up BY DP.vi"("Dew Point [DegF]"=w841, "Air Pressure [psia]"=w857, "1st known value"=w842, "1st Known Index"=w843) -> ("Output Array"=w851:dbl[])  [unwired: 11 in]
          n107 = Index Array(array=w851, index #1=0 ("index"), index #2=1 ("index"), index #3=2 ("index"), index #4=3 ("index"), index #5=4 ("index"), index #6=5 ("index")) -> (element #1=w849:dbl, element #2=w848:dbl, element #3=w847:dbl, element #4=w846:dbl, element #5=w845:dbl, element #6=w844:dbl)
        }
        frame 1 {
          # "1st Known Index"
          # "1st Known Value"
          # "KNOW: DP & WB"
          n108 = call "Psych Chart Look-up BY DP.vi"("Dew Point [DegF]"=w860, "Air Pressure [psia]"=w874, "1st known value"=w859, "1st Known Index"=w861) -> ("Output Array"=w868:dbl[])  [unwired: 11 in]
          n109 = Index Array(array=w868, index #1=0 ("index"), index #2=1 ("index"), index #3=2 ("index"), index #4=3 ("index"), index #5=4 ("index"), index #6=5 ("index")) -> (element #1=w858:dbl, element #2=w866:dbl, element #3=w865:dbl, element #4=w864:dbl, element #5=w863:dbl, element #6=w862:dbl)
        }
        frame 2 {
          # "1st Known Index"
          # "1st Known Value"
          # "KNOW: DP & RH"
          n110 = call "Psych Chart Look-up BY DP.vi"("Dew Point [DegF]"=w878, "Air Pressure [psia]"=w891, "1st known value"=w875, "1st Known Index"=w879) -> ("Output Array"=w885:dbl[])  [unwired: 11 in]
          n111 = Index Array(array=w885, index #1=0 ("index"), index #2=1 ("index"), index #3=2 ("index"), index #4=3 ("index"), index #5=4 ("index"), index #6=5 ("index")) -> (element #1=w877:dbl, element #2=w876:dbl, element #3=w883:dbl, element #4=w882:dbl, element #5=w881:dbl, element #6=w880:dbl)
        }
        frame 3 {
          # "1st Known Index"
          # "1st Known Value"
          # "KNOW: DP & HR"
          n112 = call "Psych Chart Look-up BY DP.vi"("Dew Point [DegF]"=w896, "Air Pressure [psia]"=w908, "1st known value"=w893, "1st Known Index"=w897) -> ("Output Array"=w902:dbl[])  [unwired: 11 in]
          n113 = Index Array(array=w902, index #1=0 ("index"), index #2=1 ("index"), index #3=2 ("index"), index #4=3 ("index"), index #5=4 ("index"), index #6=5 ("index")) -> (element #1=w895:dbl, element #2=w894:dbl, element #3=w892:dbl, element #4=w900:dbl, element #5=w899:dbl, element #6=w898:dbl)
        }
        frame 4 {
          # "1st Known Index"
          # "1st Known Value"
          # "KNOW: DP & Gr"
          n114 = call "Psych Chart Look-up BY DP.vi"("Dew Point [DegF]"=w914, "Air Pressure [psia]"=w925, "1st known value"=w910, "1st Known Index"=w915) -> ("Output Array"=w919:dbl[])  [unwired: 11 in]
          n115 = Index Array(array=w919, index #1=0 ("index"), index #2=1 ("index"), index #3=2 ("index"), index #4=3 ("index"), index #5=4 ("index"), index #6=5 ("index")) -> (element #1=w913:dbl, element #2=w912:dbl, element #3=w911:dbl, element #4=w909:dbl, element #5=w917:dbl, element #6=w916:dbl)
        }
        frame 5 {
          # "1st Known Index"
          # "1st Known Value"
          # "KNOW: DP & v"
          n116 = call "Psych Chart Look-up BY DP.vi"("Dew Point [DegF]"=w932, "Air Pressure [psia]"=w942, "1st known value"=w927, "1st Known Index"=w933) -> ("Output Array"=w936:dbl[])  [unwired: 11 in]
          n117 = Index Array(array=w936, index #1=0 ("index"), index #2=1 ("index"), index #3=2 ("index"), index #4=3 ("index"), index #5=4 ("index"), index #6=5 ("index")) -> (element #1=w931:dbl, element #2=w930:dbl, element #3=w929:dbl, element #4=w928:dbl, element #5=w926:dbl, element #6=w934:dbl)
        }
        frame 6 {
          # "1st Known Index"
          # "1st Known Value"
          # "KNOW: DP & h"
          n118 = call "Psych Chart Look-up BY DP.vi"("Dew Point [DegF]"=w950, "Air Pressure [psia]"=w959, "1st known value"=w943, "1st Known Index"=w951) -> ("Output Array"=w953:dbl[])  [unwired: 11 in]
          n119 = Index Array(array=w953, index #1=0 ("index"), index #2=1 ("index"), index #3=2 ("index"), index #4=3 ("index"), index #5=4 ("index"), index #6=5 ("index")) -> (element #1=w949:dbl, element #2=w948:dbl, element #3=w947:dbl, element #4=w946:dbl, element #5=w945:dbl, element #6=w944:dbl)
        }
        frame 7 {
          w960 = nan
        }
      }
    }
  }
  n120 = global read "Air Constants.vi" "Default Unknown Air State"() -> (w21:T1)
  n121 = Bundle By Name(cluster=w21, "Flow Rate [CFM]"=w10, "Pressure [psia]"=w9, "Dry Bulb Temp [DegF]"=w8, "Wet Bulb Temp [DegF]"=w7, "Relative Humidity [%]"=w6, "Humidity Ratio [lbmv/lbma]"=w5, "Grains [Gr/lbma]"=w4, "Specific Volume [ft^3/lbma]"=w3, "Enthalpy [BTU/lbm]"=w2, "Dew Point [DegF]"=w1) -> (→"Complete Air Flow State":T1)
